vi "Set Default DV.vi"(8 "error in (no error)":errorcluster, 11 "DV Default Value":i32=1000) -> (0 "error out":errorcluster)   [LabVIEW 2015]
uses:
  <vilib>/xml/Load XML File.vi
  <vilib>/xml/Close Reference(Node).vi
  <resource>/objmgr/DOMUserDefRef.rc
  <vilib>/xml/NI_XML.lvlib
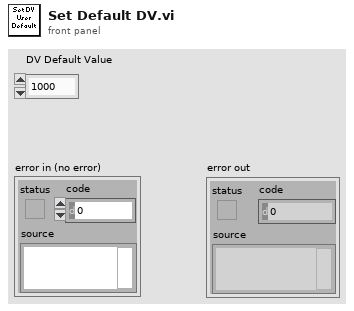
[diagram p1: front panel]
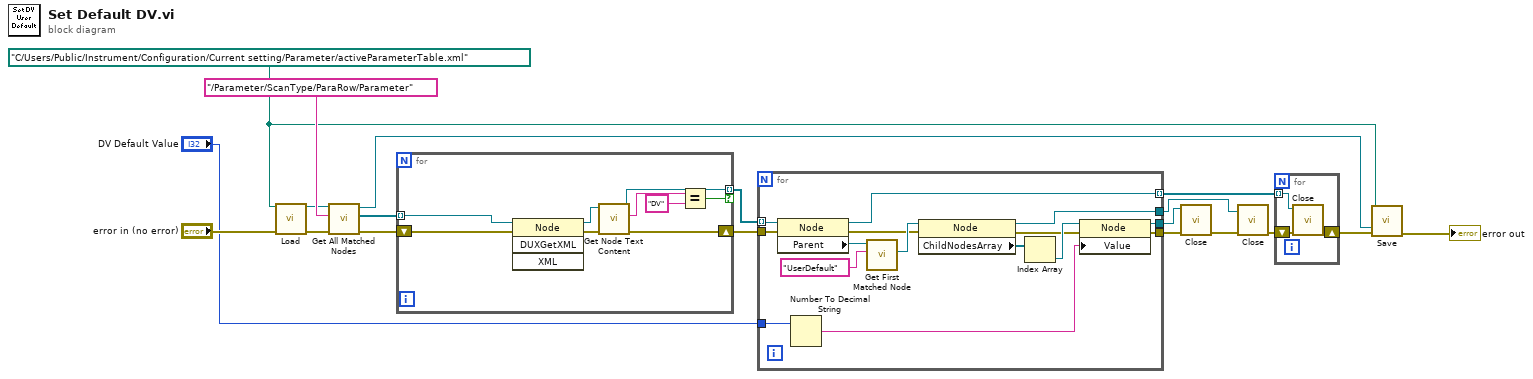
[diagram p0: block diagram]
diagram:
  w13 = path "C:/Users/Public/Instrument/Configuration/Current setting/Parameter/activeParameterTable.xml" ("Load File")
  n1 = call-poly <vilib>:"Load.vi"("path to XML document"=w13, "error in (no error)"="error in (no error)") -> ("DOM document out"=w11:refnum<k20>, "error out"=w10:errorcluster)  [unwired: 11 in, 1 out]
  n2 = call <vilib>:"Get All Matched Nodes.vi"("error in (no error)"=w10, "XPath expression"="/Parameter/ScanType/ParaRow/Parameter" ("XPath Expression"), "node in"=w11) -> ("error out"=w18:errorcluster, "node result array"=w17:refnum<k20>[], "node out"=w15:refnum<k20>)  [unwired: 6 out]
  n3 = for {
    tunnel: w17 -> [w24] mode=indexing
    shift-right: [w28] -> w12
    shift-left: w18 -> [w27]
    tunnel: [w21] -> w16 mode=indexing if=w20
    n4 = invoke on="Invoke Node" class="Node" method="DUXGetXML"(reference=w24, error in=w27) -> (reference out=w26:refnum<k20>, error out=w25:errorcluster)  [unwired: 2 in, 2 out]
    n5 = call <vilib>:"Get Node Text Content.vi"("error in (no error)"=w25, "node in"=w26) -> ("error out"=w28:errorcluster, "node text"=w22:string, "node out"=w21:refnum<k20>)  [unwired: 7 in]
    n6 = Equal?(x=w22, y="DV") -> (x = y?=w20:bool)
  }
  n7 = for {
    tunnel: w16 -> [w43] mode=indexing
    tunnel: [w32] -> w14
    tunnel: "DV Default Value" -> [w36]
    tunnel: w12 -> [w35]
    tunnel: [w31] -> w9
    tunnel: [w30] -> w8
    tunnel: [w29] -> w4 mode=indexing
    n8 = property class="Node"(reference=w43, error in=w35) -> (reference out=w29:refnum<k20>, error out=w34:errorcluster, "Parent"=w42:refnum<k20>)
    n9 = Number To Decimal String(number=w36) -> (decimal integer string=w37:string)  [unwired: 1 in]
    n10 = call <vilib>:"Get First Matched Node.vi"("XPath expression"="UserDefault", "node in"=w42) -> ("node result"=w40:refnum<k20>)  [unwired: 7 in, 2 out]
    n11 = property class="Node"(reference=w40, error in=w34) -> (reference out=w30:refnum<k20>, error out=w33:errorcluster, "ChildNodesArray"=w39:refnum<k20>[])
    n12 = Index Array(array=w39) -> (element=w38:refnum<k20>)  [unwired: 1 in]
    n13 = property class="Node"(reference=w38, error in=w33, "Value"=w37) -> (reference out=w31:refnum<k20>, error out=w32:errorcluster)
  }
  n14 = call-poly <vilib>:"Close.vi"("error in (no error)"=w14, "node"=w9) -> ("error out"=w7:errorcluster)  [unwired: 7 in]
  n15 = call-poly <vilib>:"Close.vi"("error in (no error)"=w7, "node"=w8) -> ("error out"=w6:errorcluster)  [unwired: 7 in]
  n16 = for {
    tunnel: w4 -> [w44] mode=indexing
    shift-right: [w45] -> w5
    shift-left: w6 -> [w46]
    n17 = call-poly <vilib>:"Close.vi"("error in (no error)"=w46, "node"=w44) -> ("error out"=w45:errorcluster)  [unwired: 7 in]
  }
  n18 = call <vilib>:"Save.vi"("error in (no error)"=w5, "XML file path"=w13, "DOM document in"=w15) -> ("error out"=→"error out":errorcluster)  [unwired: 6 in, 2 out]
